vi "Handle Error.vi"(8 "error in (no error)":errorcluster, 11 "IObserver in":refnum<class "IObserver.lvclass">) -> (0 "error out":errorcluster, 2 "stop actor?":bool=TRUE, 3 "IObserver out":refnum<class "IObserver.lvclass">)   [LabVIEW 2019, in "IObserver.lvlib" / "IObserver.lvclass"]
doc: "(<B>Filename</B>: Actor Framework.lvlib:Actor.lvclass:Handle Error.vi)\n\nDefines how the actor handles an error that occurred while processing a message. By default, this method does nothing except stop the actor."
uses:
  <vilib>/gpm_packages/@cs/mva-core/Source/IObserver/IObserver/IObserver.lvclass
  <vilib>/gpm_packages/@cs/event-logger/Source/Composed Log/Types/Log Level.ctl
  <vilib>/gpm_packages/@cs/mva-core/Source/IObserver/IObserver/IObserver.lvclass/IObserver.ctl
  <vilib>/gpm_packages/@cs/event-logger/Source/Composed Log/LoggerReference/LoggerReference.lvclass/LoggerReference.ctl
  <vilib>/gpm_packages/@cs/event-logger/Source/Composed Log/LoggerReference/Log Event.vi
  <vilib>/gpm_packages/@cs/event-logger/Source/Composed Log/LoggerReference/Log.vi
  <vilib>/gpm_packages/@cs/event-logger/Source/Composed Log/LoggerReference/Get Valid Event Time.vi
  <vilib>/gpm_packages/@cs/event-logger/Source/Composed Log/LoggerReference/Remove Stale Logs.vi
  <vilib>/Utility/LVClass/Get LV Class Name.vi
  <vilib>/ActorFramework/Actor/Actor.lvclass
  <vilib>/gpm_packages/@cs/event-logger/Source/Composed Log/Composed Log.lvlib
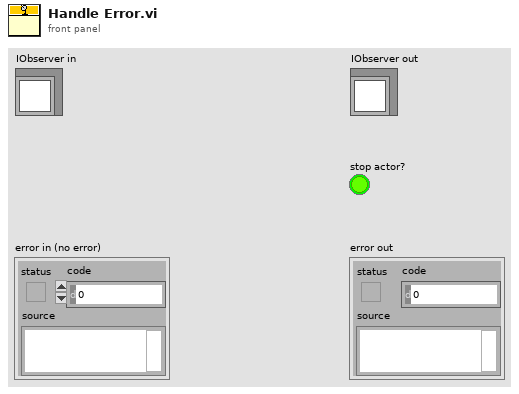
[diagram p1: front panel]
types:
  T1 = typedef "Composed Log.lvlib/Log Level.ctl" = enum16{"Debug", "Info", "Warning", "Error", "Critical"}
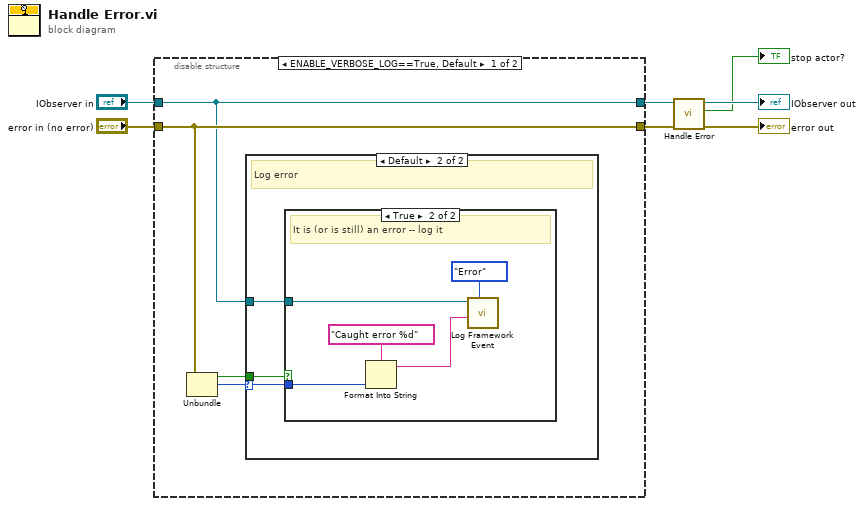
[diagram p0: block diagram]
diagram:
  n1 = disable-structure shown="ENABLE_VERBOSE_LOG==True, Default" {
    disable-tunnel: "IObserver in" -> [w10 w21]
    disable-tunnel: [w10 w21] -> w2
    disable-tunnel: "error in (no error)" -> [w11 w20]
    disable-tunnel: [w11 w20] -> w1
    frame condition #0 (active) {
      # "Log caught errors by default"
      n2 = Unbundle(w11) -> ("status"=w8:bool, "code"=w9:i32)  [unwired: 1 out]
      n3 = case shown="Default" w9 {
        selector: w9 -> [_ w14]
        tunnel: w10 -> [_ w13]
        tunnel: w8 -> [_ w12]
        frame 43, 1608 {
          # "Actor shutdown error -- Do not log"
        }
        frame Default {
          # "Log error"
          n4 = case shown="True" w12 {
            tunnel: w14 -> [_ w18]
            tunnel: w13 -> [_ w17]
            frame False {
              # "Assume the one who cleared it\ntook care of business properly."
              # "Must have been cleared!"
            }
            frame True {
              # "It is (or is still) an error -- log it"
              n5 = Format Into String(format string="Caught error %d", w18) -> (resulting string=w15:string)  [unwired: 2 in, 1 out]
              n6 = call <vilib>:"Log Framework Event.vi"("Event Level (Debug)"=Log_Level."Error", "Data To Log"=w15, "IObserver in"=w17) -> ()  [unwired: 8 in, 1 out]
            }
          }
        }
      }
    }
    frame condition #1 {
      # "Remove all logging from this method at compile time"
    }
  }
  n7 = call-parent "Handle Error.vi"("error in (no error)"=w1, "Actor in"=w2) -> ("error out"=→"error out":errorcluster, "stop actor?"=→"stop actor?":bool, "Actor out"=→"IObserver out":refnum<class "IObserver.lvclass">)  [unwired: 7 in]
